vi "Receive Message.vi"(6 "priority":i32, 10 "IObserver in":refnum<class "IObserver.lvclass">, 11 "Message in":refnum<class "Message.lvclass">) -> (0 "error out":errorcluster, 2 "Actor out":refnum<class "Actor.lvclass">)   [LabVIEW 2017, in "IObserver.lvlib" / "IObserver.lvclass"]
doc: "This VI should be overriden ONLY if you are creating a proxy actor for remote transmission. If you are, override this VI to transmit the received message to a new destination, maintaining the given priority."
uses:
  IObserver.lvclass
  Transport/ActorMessageTransport/Notification Msg/Notification Msg.lvclass
  IObserver Messages/Observe Data Msg/Observe Data Msg.lvclass
  <vilib>/ActorFramework/Actor/Actor.lvclass
  gpm_packages/@cs/actor-framework-messages/Source/MessageCycle/MessageCycle.lvclass
  gpm_packages/@cs/event-logger/Source/Composed Log/Types/Log Level.ctl
  gpm_packages/@cs/event-logger/Source/Composed Log/Composed Log.lvlib
  <vilib>/ActorFramework/Message/Message.lvclass
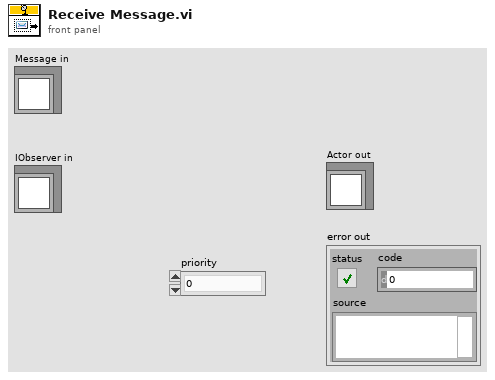
[diagram p1: front panel]
types:
  T1 = typedef "Composed Log.lvlib/Log Level.ctl" = enum16{"Debug", "Info", "Warning", "Error", "Critical"}
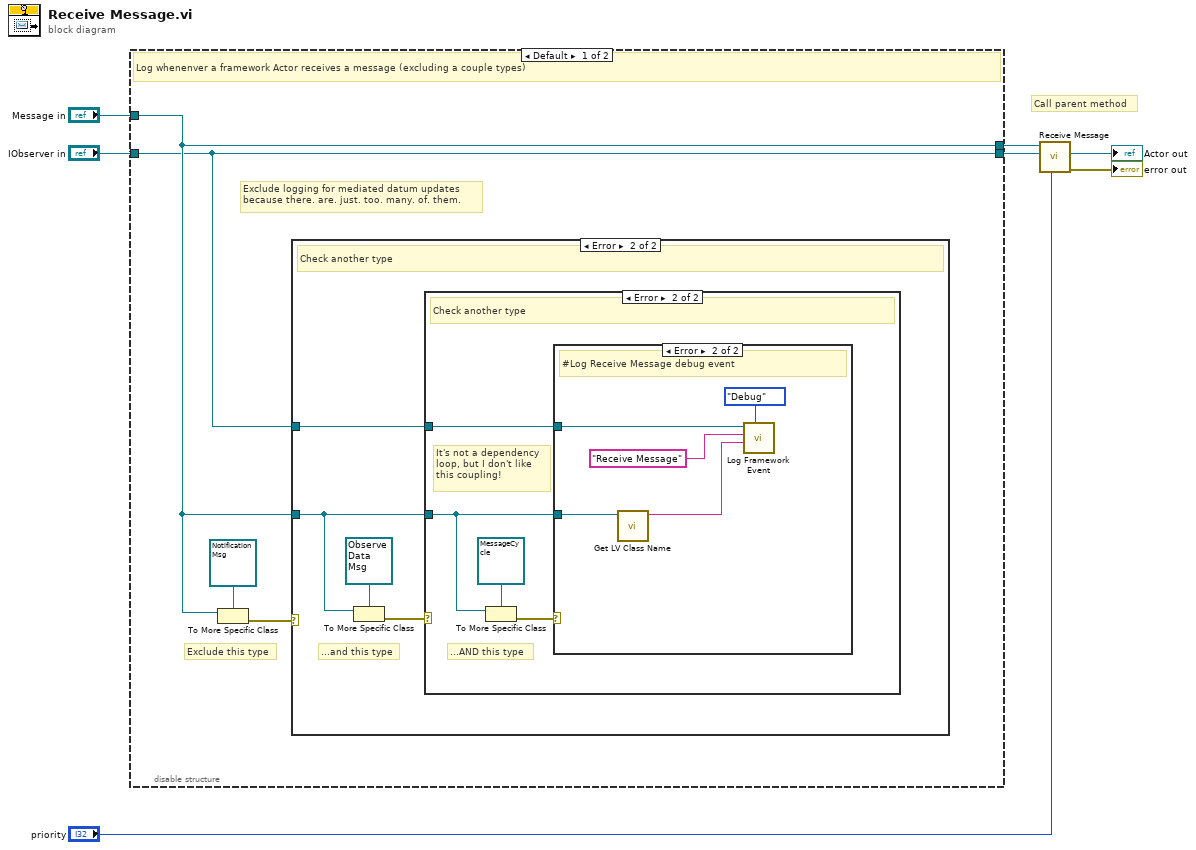
[diagram p0: block diagram]
diagram:
  # "Call parent method"
  n1 = disable-structure shown="Default" {
    disable-tunnel: "Message in" -> [w9 w26]
    disable-tunnel: "IObserver in" -> [w8 w25]
    disable-tunnel: [w9 w26] -> w2
    disable-tunnel: [w8 w25] -> w1
    frame condition #0 (active) {
      # "Exclude this type"
      # "Exclude logging for mediated datum updates\nbecause there. are. just. too. many. of. them."
      # "Log whenenver a framework Actor receives a message (excluding a couple types)"
      n2 = To More Specific Class(target class=refnum<class "Notification Msg.lvclass"> refnum ("Transport.lvlib:Notification Msg.lvclass"), reference=w9) -> (error out=w10:errorcluster)  [unwired: 1 in, 1 out]
      n3 = case shown="Error" w10 {
        tunnel: w9 -> [_ w13]
        tunnel: w8 -> [_ w12]
        frame No Error {
          # "Message is a descendant of Notification Msg -- Do not log this message type"
        }
        frame Error {
          # "...and this type"
          # "Check another type"
          n4 = To More Specific Class(target class=refnum<class "Observe Data Msg.lvclass"> refnum ("IObserver.lvlib:Observe Data Msg.lvclass"), reference=w13) -> (error out=w14:errorcluster)  [unwired: 1 in, 1 out]
          n5 = case shown="Error" w14 {
            tunnel: w13 -> [_ w17]
            tunnel: w12 -> [_ w19]
            frame No Error {
              # "Message is a descendant of Observe Data Msg -- Do not log"
            }
            frame Error {
              # "It's not a dependency\nloop, but I don't like\nthis coupling!"
              # "...AND this type"
              # "Check another type"
              n6 = To More Specific Class(target class=refnum<class "MessageCycle.lvclass"> refnum ("MessageCycle.lvclass"), reference=w17) -> (error out=w16:errorcluster)  [unwired: 1 in, 1 out]
              n7 = case shown="Error" w16 {
                tunnel: w19 -> [_ w23]
                tunnel: w17 -> [_ w20]
                frame No Error {
                  # "Doh... Don't log this type either."
                }
                frame Error {
                  # "#Log Receive Message debug event"
                  n8 = call <vilib>:"Get LV Class Name.vi"("object"=w20) -> ("class name"=w21:string)  [unwired: 9 in, 1 out]
                  n9 = call "Log Framework Event.vi"("Event Level (Debug)"=Log_Level."Debug", "Data To Log"=w21, "Caller Info (\"\")"="Receive Message" ("Caller Info (\"\")"), "IObserver in"=w23) -> ()  [unwired: 7 in, 1 out]
                }
              }
            }
          }
        }
      }
    }
    frame condition #1 {
      # "Remove all logging from this method at compile time"
    }
  }
  n10 = call-parent "Receive Message.vi"("priority"="priority", "Actor in"=w1, "Message in"=w2) -> ("error out"=→"error out":errorcluster, "Actor out"=→"Actor out":refnum<class "Actor.lvclass">)  [unwired: 7 in]
